vi "SRV_Sensor View Tab_Set Captions.vi"(5 "Sensor View refs":T7, 7 "Sensors Config":T1[](array[typedef]) {"Register" format="%.0x"; "I2C Address" format="%.0x"; "Sample Period (ms)" min=10 max=60000 step=1; "Digital Mask" format="%.0x"; "Channel" format="%.0x"}, 11 "error in (no error)":errorcluster) -> (6 "Sensor View refs dup":T7, 15 "error out":errorcluster)   [LabVIEW 2009]
uses:
  SRV_Sensor View refs.ctl
  SRV_Sensor Config Cluster.ctl
  SRV_Sensor Analog-Digital.ctl
  SRV_Sensor Sampling Mode.ctl
  SRV_Sensor View Config Cluster.ctl
  SRV_Sensors Names.ctl
  SRV_Sensor PicoC Shared Var Type.ctl
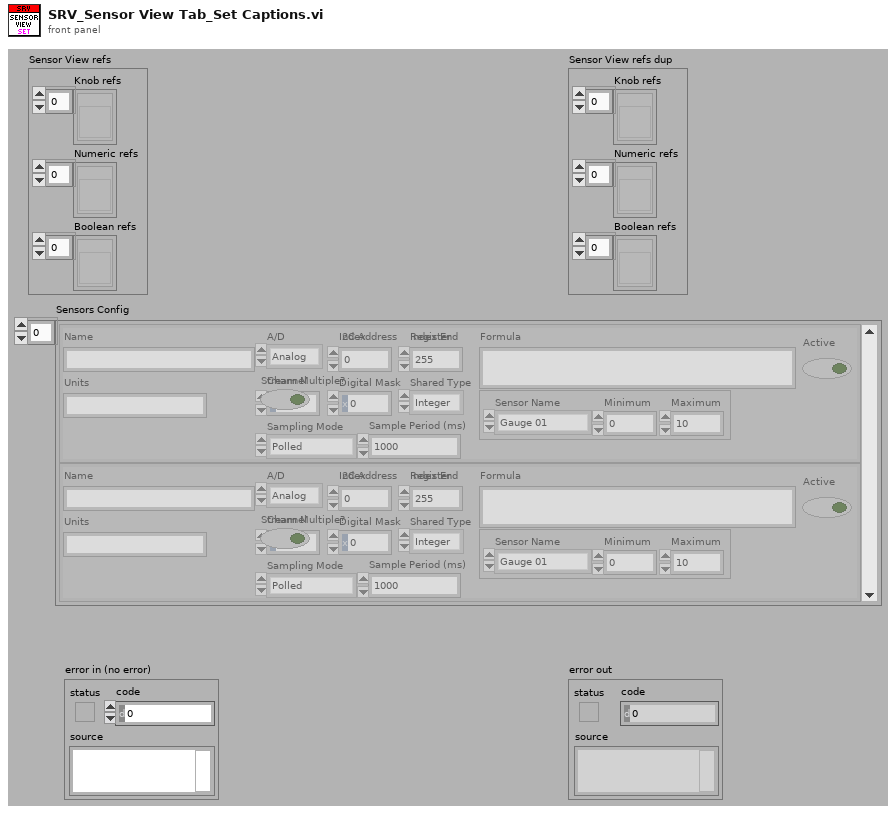
[diagram p1: front panel]
types:
  T1 = typedef "SRV_Sensor Config Cluster.ctl" = cluster{"Name":string, "A/D":T2, "I2C Address":u8, "Register":u8, "Channel":u8, "Digital Mask":u8, "Units":string, "Sampling Mode":T3, "Sample Period (ms)":u32, "Formula":string, "Sensor View Config":T4, "Active":bool, "PicoC Shared Var Type":T6, "Index":u8, "Stream Multiple?":bool, "Index End":u8}
  T2 = typedef "SRV_Sensor Analog-Digital.ctl" = enum16{"Analog", "Digital", "RCMx1 Analog", "PicoC Shared"}
  T3 = typedef "SRV_Sensor Sampling Mode.ctl" = enum16{"Polled", "Streaming"}
  T4 = typedef "SRV_Sensor View Config Cluster.ctl" = cluster{"Sensor Name":T5, "Minimum":dbl, "Maximum":dbl}
  T5 = typedef "SRV_Sensors Names.ctl" = enum16{"Gauge 01", "Gauge 02", "Gauge 03", "Gauge 04", "Meter 01", "Meter 02", "Meter 03", "Meter 04", "Numeric 01", "Numeric 02", "Numeric 03", "Numeric 04", "Numeric 05", "Numeric 06", "Numeric 07", "Numeric 08", "Boolean 01", "Boolean 02", "Boolean 03", "Boolean 04", "Boolean 05", "Boolean 06", "Boolean 07", "Boolean 08", "Boolean 09", "Boolean 10", "Boolean 11", "Boolean 12", "Boolean 13", "Boolean 14", "Boolean 15", "Boolean 16", "Boolean 17", "Boolean 18", "Boolean 19", "Boolean 20", "Boolean 21", "Boolean 22", "Boolean 23", "Boolean 24", "Boolean 25", "Boolean 26", "Boolean 27", "Boolean 28", "Boolean 29", "Boolean 30", "Boolean 31", "Boolean 32"}
  T6 = typedef "SRV_Sensor PicoC Shared Var Type.ctl" = enum16{"String", "Integer", "Float"}
  T7 = typedef "SRV_Sensor View refs.ctl" = cluster{"Knob refs":refnum<vi>[], "Numeric refs":refnum<vi>[], "Boolean refs":refnum<vi>[]}
  T8 = enum8{"Enabled", "Disabled", "Disabled and Grayed Out"}
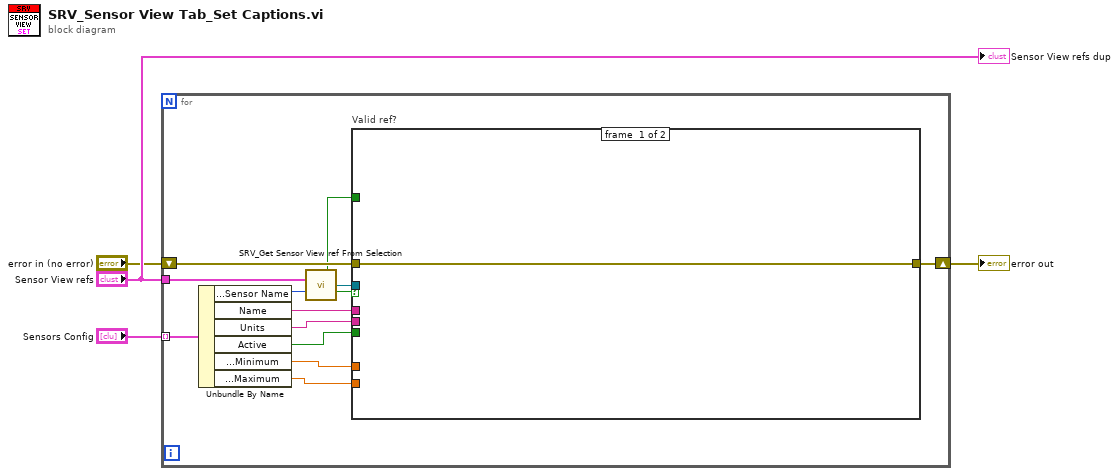
[diagram p0: block diagram]
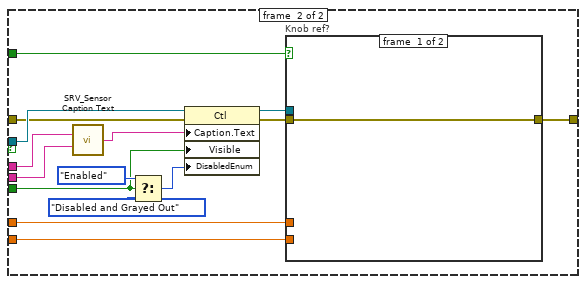
[diagram p2: hidden frame]
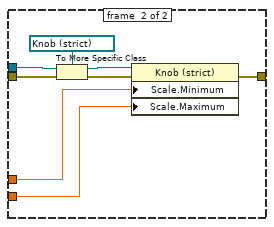
[diagram p3: hidden frame]
diagram:
  n1 = for {
    tunnel: "Sensors Config" -> [w17] mode=indexing
    tunnel: "Sensor View refs" -> [w15]
    shift-right: [w8] -> w1
    shift-left: "error in (no error)" -> [w12]
    n2 = Unbundle By Name(w17) -> ("Sensor View Config.Sensor Name"=w16:T5, "Name"=w13:string, "Units"=w5:string, "Active"=w10:bool, "Sensor View Config.Minimum"=w9:dbl, "Sensor View Config.Maximum"=w7:dbl)
    n3 = call "SRV_Get Sensor View ref From Selection.vi"("Sensor View refs"=w15, "Sensor View"=w16) -> ("Knob ref?"=w6:bool, "Selected ref"=w14:refnum<vi>, "Valid ref?"=w11:bool)  [unwired: 9 in, 2 out]
    n4 = case "Valid ref?" shown="True" w11 {
      tunnel: w14 -> [_ w33]
      tunnel: w13 -> [_ w21]
      tunnel: w12 -> [w18 w32]
      tunnel: [w18 w30] -> w8
      tunnel: w6 -> [_ w29]
      tunnel: w10 -> [_ w23]
      tunnel: w9 -> [_ w27]
      tunnel: w7 -> [_ w26]
      tunnel: w5 -> [_ w20]
      frame #0 {
      }
      frame #1 {
        n5 = call "SRV_Sensor Caption Text.vi"("Name"=w21, "Units"=w20) -> ("Sensor Caption Text"=w19:string)  [unwired: 13 in]
        n6 = Select(t=T8."Enabled" ("Disabled"), s=w23, f=T8."Disabled and Grayed Out" ("Disabled")) -> (s? t:f=w22:T8)
        n7 = property class="Ctl"(reference=w33, error in=w32, "Caption.Text"=w19, "Visible"=w23, "DisabledEnum"=w22) -> (reference out=w28:refnum<vi>, error out=w31:errorcluster)
        n8 = case "Knob ref?" shown="True" w29 {
          tunnel: w31 -> [w34 w39]
          tunnel: [w34 w42] -> w30
          tunnel: w28 -> [_ w37]
          tunnel: w27 -> [_ w35]
          tunnel: w26 -> [_ w36]
          frame #0 {
          }
          frame #1 {
            n9 = To More Specific Class(target class=refnum<vi> refnum ("Meter 04"), reference=w37, error in=w39) -> (specific class reference=w40:refnum<vi>, error out=w38:errorcluster)
            n10 = property class="Knob (strict)"(reference=w40, error in=w38, "Scale.Minimum"=w35, "Scale.Maximum"=w36) -> (error out=w42:errorcluster)  [unwired: 1 out]
          }
        }
      }
    }
  }
  "error out" <- w1
  "Sensor View refs dup" <- "Sensor View refs"
